vi "JKISM++ Send Message and Wait for Reply.vi"(6 "Response Timeout(5000ms)":i32=5000, 8 "Error In (no error)":errorcluster, 9 "Target Module":string="A", 10 "Arguments (\"\")":string, 11 "State":string="DoA") -> (0 "error out":errorcluster, 2 "Arguments":string="DoA")   [LabVIEW 2014, in "JKI State Machine++.lvlib"]
doc: "Send a message to JKISM specified and wait for the reply with timeout.\n\n<b>Inputs:</b>\n - <b>Target Module</b>: Target JKISM Module name.\n - <b>State</b>: Message to send\n - <b>Arguments (\"\")</b>: Argument of the message.\n - <b>Response Timeout(5000ms)</b>: Timeout for waiting the response.\n - <b>Error In (no error)</b>: Error cluster\n\n<b>Outputs:</b>\n - <b>Arguments</b>: Response returned.\n - <b>error out</b>: Error cluster"
uses:
  JKI State Machine++.lvlib
  _Support/JKISMQ/_Obtain JKISMQ.vi
  _Support/FGV-BroadcastRegistry/Cache-Broadcast Registry Search Result.vi
  _Support/JKISMQ/_Create Resp Queue.vi
  _Support/JKISMQ/_Unlock JKISMQ.vi
  _Support/JKISMQ/_Lock State JKISMQ.vi
  _Support/JKISMQ/_Release JKISMQ.vi
  _Support/JKISMQ/_Input Name to JKISM Mode.vi
  _Support/GlobalEvent/FGV-GlobalEventRef.vi
  _Support/JKISMQ/_JKISMQFGV.vi
  _Support/JKISMQ/_Enqueue JKISMQ.vi
  _Support/FGV-BroadcastRegistry/global-JKISMQ FGV Change Flag.vi
  _Support/FGV-BroadcastRegistry/FGV-BroadcastRegistry.vi
  _Support/FGV-BroadcastRegistry/global-Broadcast Cache Change Flag.vi
  _Support/JKISMQ/_Dequeue JKISMQ.vi
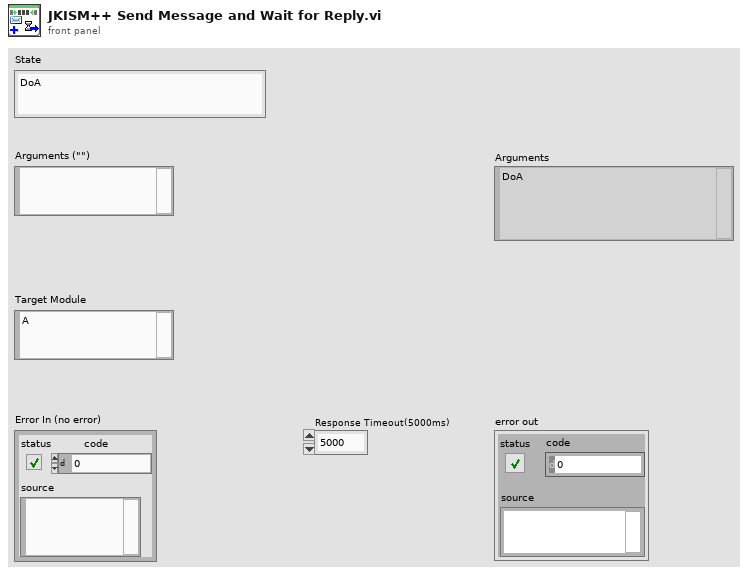
[diagram p1: front panel]
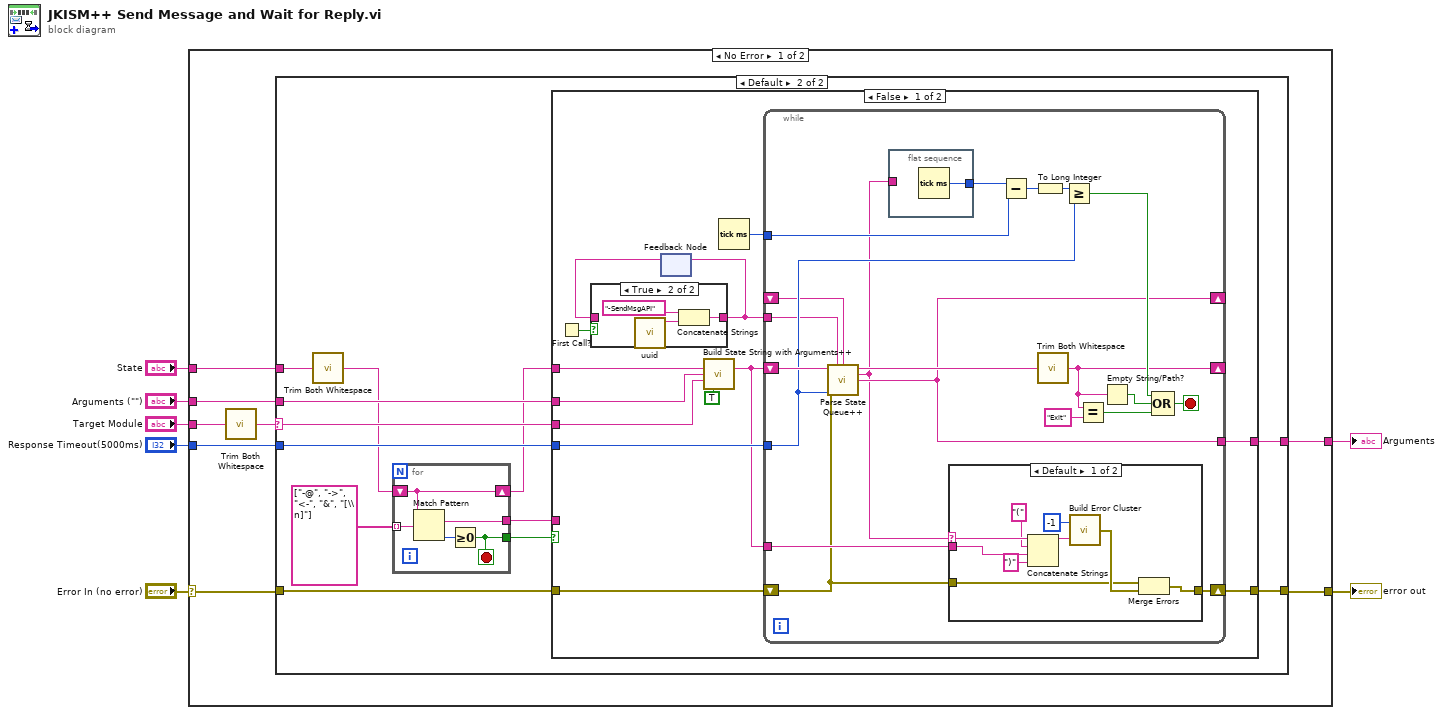
[diagram p0: block diagram]
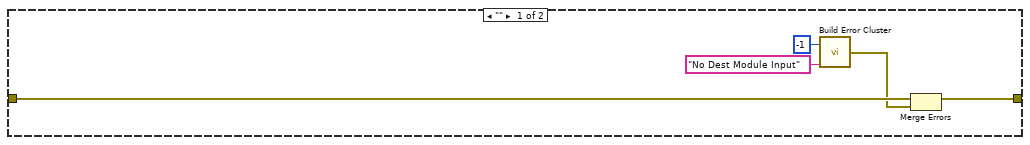
[diagram p2: hidden frame]
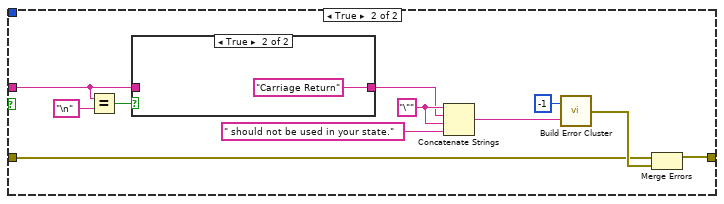
[diagram p5: hidden frame]
diagram:
  n1 = case shown="No Error" "Error In (no error)" {
    selector: "Error In (no error)" -> [w14 w99]
    tunnel: "State" -> [w15 _]
    tunnel: "Response Timeout(5000ms)" -> [w13 _]
    tunnel: [w9 w99] -> w4
    tunnel: [w12 _] -> w3
    tunnel: "Target Module" -> [w11 _]
    tunnel: "Arguments (\"\")" -> [w10 _]
    frame No Error {
      n2 = call "Trim Both Whitespace.vi"("string"=w11) -> ("trimmed string"=w8:string)  [unwired: 1 in]
      n3 = case shown="Default" w8 {
        selector: w8 -> [_ w29]
        tunnel: w14 -> [w18 w32]
        tunnel: w13 -> [_ w31]
        tunnel: [_ w30] -> w12
        tunnel: w10 -> [_ w28]
        tunnel: [w17 w27] -> w9
        tunnel: w15 -> [_ w26]
        frame "" {
          n4 = call "Build Error Cluster.vi"("String to Prepend to source (\"\")"="No Dest Module Input" ("String to Prepend to source (\"\")"), "code"=-1) -> ("error out"=w16:errorcluster)
          n5 = Merge Errors(w18, w16) -> (w17:errorcluster)
        }
        frame Default {
          n6 = call "Trim Both Whitespace.vi"("string"=w26) -> ("trimmed string"=w21:string)  [unwired: 1 in]
          n7 = for {
            shift-right: [w98] -> w25
            shift-left: w21 -> [w98]
            tunnel: string[] ["-@", "->", "<-", "&", "[\\n]"] -> [w97] mode=indexing
            tunnel: [w95] -> w23
            tunnel: [w94] -> w24
            stop <- w94 stop-if-true
            n8 = Match Pattern(string=w98, regular expression=w97) -> (match substring=w95:string, offset past match=w96:i32)  [unwired: 1 in, 2 out]
            n9 = Greater Or Equal To 0?(x=w96) -> (x >= 0?=w94:bool)
          }
          n10 = case shown="False" w24 {
            tunnel: w32 -> [w45 w87]
            tunnel: w31 -> [w44 _]
            tunnel: [w42 _] -> w30
            tunnel: w29 -> [w40 _]
            tunnel: w28 -> [w39 _]
            tunnel: [w38 w88] -> w27
            tunnel: w25 -> [w33 _]
            tunnel: w23 -> [_ w83]
            frame False {
              n11 = First Call?() -> (First Call?: T/F=w35:bool)
              n12 = feedback #1() -> (w34:string)  [unwired: 1 in]
              n13 = case shown="True" w35 {
                tunnel: [w46 w47] -> w36
                tunnel: w34 -> [w46 _]
                frame False {
                }
                frame True {
                  n14 = call "uuid.vi"() -> ("UUID"=w48:string)  [unwired: 11 in]
                  n15 = Concatenate Strings("-SendMsgAPI" ("Name(\"\" to use uuid)"), w48) -> (w47:string)
                }
              }
              n16 = feedback-in #1(w36) -> ()
              n17 = call "Build State String with Arguments++.vi"("State"=w33, "Arguments (\"\")"=w39, "Target Module (\"\")"=w40, "Sync-Call(-@) T By Default/Async-Call(->) F"=TRUE ("Sync-Call(@) T By Default/Async-Call(->) F")) -> ("State with Arguments"=w37:string)  [unwired: 11 in]
              n18 = Tick Count (ms)() -> (millisecond timer value=w43:u32)
              n19 = while {
                shift-right: [w50] -> _
                shift-left: w37 -> [w69]
                tunnel: w44 -> [w63]
                tunnel: w43 -> [w66]
                tunnel: [w60] -> w42
                shift-right: [w60] -> _
                shift-left: _ -> [w59]
                tunnel: w36 -> [w58]
                tunnel: w37 -> [w56]
                shift-right: [w55] -> w38
                shift-left: w45 -> [w54]
                stop <- w65 stop-if-true
                n20 = call "Parse State Queue++.vi"("State Queue"=w69, "Name(\"\" to use uuid)"=w58, "Response Arguments"=w59, "Error In (no error)"=w54, "Response Timeout(5000ms)"=w63) -> ("Remaining States"=w68:string, "Current State"=w57:string, "Arguments"=w60:string)  [unwired: 5 in, 3 out]
                n21 = flat-sequence {
                  tunnel: [w80] -> w67
                  tunnel: w57 -> [_]
                  frame #0 {
                    n22 = Tick Count (ms)() -> (millisecond timer value=w80:u32)
                  }
                }
                n23 = case shown="Default" w57 {
                  selector: w57 -> [w77 _]
                  tunnel: [w74 w79] -> w55
                  tunnel: w54 -> [w73 w79]
                  tunnel: w56 -> [w72 _]
                  frame Default {
                    n24 = Concatenate Strings(w77, "(" ("string"), w72, ")" ("string")) -> (w76:string)
                    n25 = call "Build Error Cluster.vi"("String to Prepend to source (\"\")"=w76, "code"=-1) -> ("error out"=w75:errorcluster)
                    n26 = Merge Errors(w73, w75) -> (w74:errorcluster)
                  }
                  frame "Response" {
                  }
                }
                n27 = Subtract(x=w67, y=w66) -> (x-y=w64:u32)
                n28 = To Long Integer(number=w64) -> (32bit integer=w61:i32)
                n29 = call "Trim Both Whitespace.vi"("string"=w68) -> ("trimmed string"=w50:string)  [unwired: 1 in]
                n30 = Greater Or Equal?(x=w61, y=w63) -> (x >= y?=w62:bool)
                n31 = Equal?(x=w50, y="Exit" ("State(s) at Back (\"\")")) -> (x = y?=w53:bool)
                n32 = Empty String/Path?(string/path=w50) -> (empty?=w51:bool)
                n33 = Compound Arithmetic op=OR(w62, w51, w53) -> (w65:bool)
              }
            }
            frame True {
              w85 = "\"" ("string")
              n34 = Equal?(x=w83, y="\n" ("regular expression")) -> (x = y?=w81:bool)
              n35 = case shown="True" w81 {
                tunnel: [w92 "Carriage Return" ("State")] -> w84
                tunnel: w83 -> [w92 _]
                frame False {
                }
                frame True {
                }
              }
              n36 = Concatenate Strings(w85, w84, w85, " should not be used in your state." ("String to Prepend to source (\"\")")) -> (w86:string)
              n37 = call "Build Error Cluster.vi"("String to Prepend to source (\"\")"=w86, "code"=-1) -> ("error out"=w89:errorcluster)
              n38 = Merge Errors(w87, w89) -> (w88:errorcluster)
            }
          }
        }
      }
    }
    frame Error {
    }
  }
  "error out" <- w4
  "Arguments" <- w3
